vi "GenWhiteKeyDataArray.vi"(7 "WhiteKeySize":cluster{"Width":i32, "Hieght":i32}={"Width"=21, "Hieght"=147}, 8 "error in (no error)":errorcluster) -> (0 "error out":errorcluster, 2 "WhiteKeyData array":u32[][](array[numeric]))   [LabVIEW 2015]
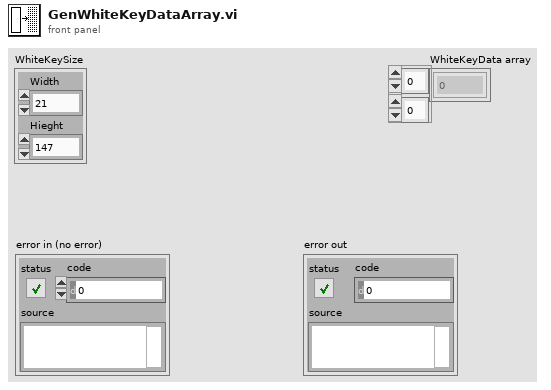
[diagram p1: front panel]
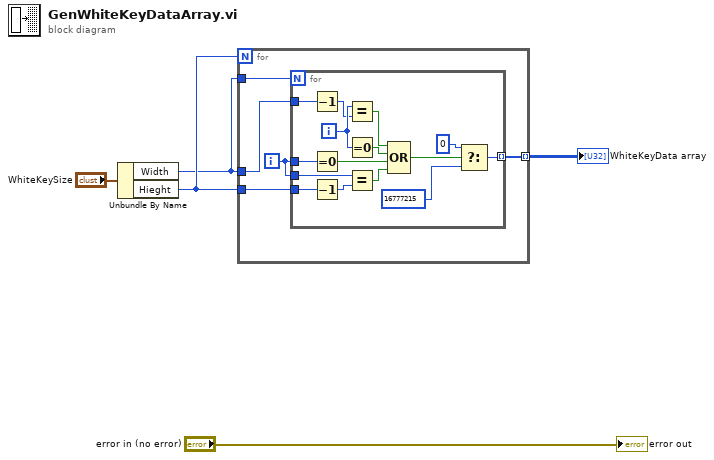
[diagram p0: block diagram]
diagram:
  n1 = Unbundle By Name("WhiteKeySize") -> ("Width"=w3:i32, "Hieght"=w4:i32)
  n2 = for {
    N: w4 -> [_]
    tunnel: w3 -> [w8]
    tunnel: w4 -> [w9]
    tunnel: [w10] -> w2 mode=indexing
    tunnel: w3 -> [w6]
    i -> [w7]
    n3 = for {
      N: w6 -> [_]
      tunnel: [w22] -> w10 mode=indexing
      tunnel: w7 -> [w21]
      tunnel: w9 -> [w11]
      tunnel: w8 -> [w15]
      tunnel: w7 -> [w13]
      i -> [w25]
      n4 = Decrement(x=w15) -> (x-1=w14:i32)
      n5 = Equal To 0?(x=w21) -> (x = 0?=w18:bool)
      n6 = Decrement(x=w11) -> (x-1=w12:i32)
      n7 = Equal?(x=w25, y=w14) -> (x = y?=w20:bool)
      n8 = Equal To 0?(x=w25) -> (x = 0?=w19:bool)
      n9 = Equal?(x=w13, y=w12) -> (x = y?=w17:bool)
      n10 = Compound Arithmetic op=OR(w20, w19, w18, w17) -> (w16:bool)
      n11 = Select(t=u32 0, s=w16, f=u32 16777215) -> (s? t:f=w22:u32)
    }
  }
  "WhiteKeyData array" <- w2
  "error out" <- "error in (no error)"
